vi "TA_Index_Time.vi.vi"(10 "Selected Time":dbl[](array[numeric])=[0.324, 0.47, 0.67, 2.02, 5.03, 32.2, 100.0, 220.0, 440.0, 1000.0], 11 "Time (ps)":dbl[](array[numeric])=[-8.76278115, -7.76208066, -6.76138017, -5.76067968, -4.78666453, -3.78596404, -2.78526355, -1.78456306, -0.783862574, -0.717149208, -0.677121189, -0.623750496, -0.583722476, -0.530351783, -0.476981091, -0.436953071, -0.383582378, -0.330211685, -0.276840993, -0.236812973, -0.18344228, -0.130071587, -0.0767008946, -0.0366728746, 0.0166978184, 0.0700685114, 0.123439204, 0.163467224, 0.216837916, 0.270208609, 0.323579302, 0.363607321, 0.430320687, 0.470348707, 0.5237194, 0.563747419, 0.617118112, 0.670488805, 0.723859498, 0.763887517, 0.81725821, 0.870628903, 0.923999596, 0.964027615, 1.03074098, 1.070769, 1.12413969, 1.16416771, 1.21753841, 1.33762247, 1.41767851, 1.53776257, 1.61781861, 1.73790267, 1.8179587, 1.93804276, 2.0180988, 2.13818286, 2.2182389, 2.418379, 2.6185191, 2.83200187, 3.03214197, 3.23228206, 3.43242216, 3.61921959, 3.83270236, 4.01949978, 4.21963988, 4.43312265, 4.63326275, 4.82006018, 5.03354295, 5.22034037, 5.71401928, 6.22104086, 6.71471977, 7.22174135, 7.71542026, 8.22244184, 8.71612075, 9.22314233, 9.71682124, 10.2238428, 11.2245433, 12.2252438, 13.2259443, 14.2133021, 15.2140026, 16.2147031, 17.2287462, 18.2294467, 19.2301472, 20.2308477, 22.218906, 24.220307, 26.221708, 28.2364516, 30.2245099, 32.2392536, 34.2139692, 36.2287129, 38.2301139, 40.2181722, 42.2195731, 44.2343168, 46.2223751, 48.2371188, 50.2251771, 55.2153368, 60.2188393, 65.2223418, 70.2258442, 75.216004, 80.2195064, 85.2230089, 90.2131687, 95.2166711, 100.220174, 110.213836, 120.220841, 130.214503, 140.221508, 150.21517, 160.222175, 170.215837, 180.222842, 190.216504, 200.223509, 220.210834, 240.224844, 260.212168, 280.226178, 300.213502, 320.200827, 340.201494, 360.215504, 380.216171, 400.216838, 420.204162, 440.218172, 460.205497, 480.206164, 500.206831, 550.201827, 600.210167, 650.205163, 700.20016, 750.208499, 800.203495, 850.211834, 900.206831, 950.201827, 1000.21017]) -> (3 "Index of Selected Time":i32[](array[numeric]))   [LabVIEW 2025]
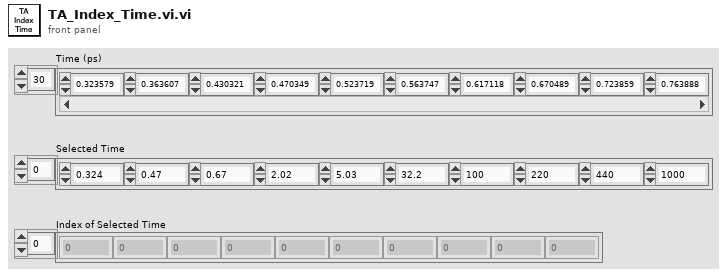
[diagram p1: front panel]
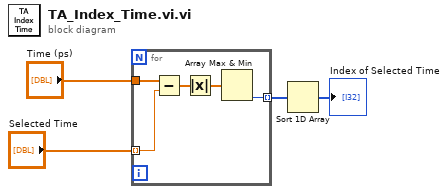
[diagram p0: block diagram]
diagram:
  n1 = for {
    tunnel: "Time (ps)" -> [w9]
    tunnel: "Selected Time" -> [w8] mode=indexing
    tunnel: [w5] -> w2 mode=indexing
    n2 = Subtract(x=w9, y=w8) -> (x-y=w7:dbl[])
    n3 = Absolute Value(x=w7) -> (abs(x)=w6:dbl[])
    n4 = Array Max & Min(array=w6) -> (min index (indices)=w5:i32)  [unwired: 3 out]
  }
  n5 = Sort 1D Array(array=w2) -> (sorted array=→"Index of Selected Time":i32[])
